vi "Lidar send UDP Frame.vi"(10 "reference":refnum<vi>, 11 "Notifier in":refnum<notifier>) -> (0 "error out":errorcluster)   [LabVIEW 2015]
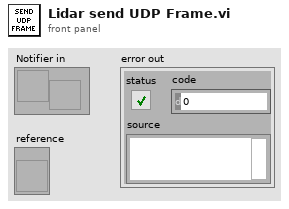
[diagram p1: front panel]
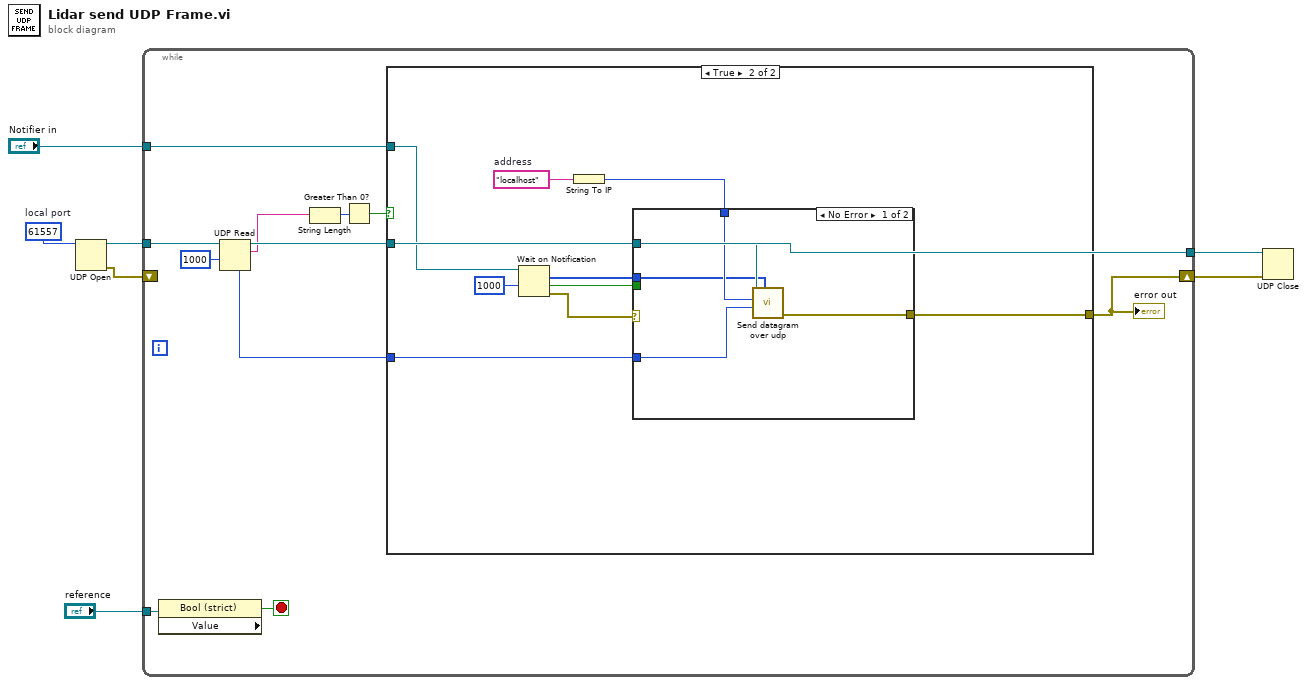
[diagram p0: block diagram]
diagram:
  w2 = u16 61557  # local port
  n1 = UDP Open(11:w2) -> (port=w4:refnum<k16>, 0:w6:errorcluster)  [unwired: 4 in, 1 out]
  n2 = while {
    tunnel: "Notifier in" -> [w9]
    tunnel: w4 -> [w17]
    tunnel: [w16] -> w5
    shift-right: [w18] -> w7
    shift-left: w6 -> [_]
    tunnel: "reference" -> [w8]
    stop <- w12 stop-if-true
    n3 = property class="Bool (strict)"(reference=w8) -> ("Value"=w12:bool)  [unwired: 1 in, 2 out]
    n4 = UDP Read(connection ID=w17, timeout ms (25000)=1000) -> (data out=w14:string, 3:w16:refnum<k16>, 4:w11:u16)  [unwired: 2 in, 2 out]
    n5 = String Length(string=w14) -> (length=w13:i32)
    n6 = Greater Than 0?(x=w13) -> (x > 0?=w10:bool)
    n7 = case shown="True" w10 {
      tunnel: w16 -> [_ w26]
      tunnel: [_ w25] -> w18
      tunnel: w11 -> [_ w24]
      tunnel: w9 -> [_ w23]
      frame False {
      }
      frame True {
        w27 = "localhost"  # address
        n8 = Wait on Notification(notifier=w23, timeout in ms (-1)=1000) -> (notification=w22:u32[], timed out?=w19:bool, error out=w20:errorcluster)  [unwired: 2 in, 1 out]
        n9 = String To IP(1:w27) -> (0:w28:u32)
        n10 = case shown="No Error" w20 {
          selector: w20 -> [_ w34]
          tunnel: w28 -> [w33 _]
          tunnel: w26 -> [w32 _]
          tunnel: [w31 w34] -> w25
          tunnel: w24 -> [w30 _]
          tunnel: w22 -> [w29 _]
          tunnel: w19 -> [_ _]
          frame No Error {
            n11 = call "Send datagram over udp.vi"("Data"=w29, "port"=w30, "Address"=w33, "IDP ref"=w32) -> ("error out"=w31:errorcluster)  [unwired: 7 in]
          }
          frame Error {
          }
        }
      }
    }
    "error out" <- w18
  }
  n12 = UDP Close(connection ID=w5, 8:w7) -> ()  [unwired: 2 out]
